vi "lfieldpanel_plot_sensor_data.vi"(7 "Integrate":bool, 8 "error in (no error)":errorcluster, 9 "First_time?":bool, 10 "image_data":T1, 11 "lightfield_panel in":refnum<class "lightfield_panel.lvclass">) -> (0 "error out":errorcluster, 3 "lightfield_panel out":refnum<class "lightfield_panel.lvclass">)   [LabVIEW 2015, in "lightfield_panel.lvclass"]
uses:
  lightfield_panel.lvclass
  UI/panel_class/panel.lvclass/panel.ctl
  <vilib>/Analysis/1siggen.llb/Ramp Pattern by Samples.vi
  UI/panel_class/panel.lvclass
  <vilib>/Analysis/NI_AALBase.lvlib
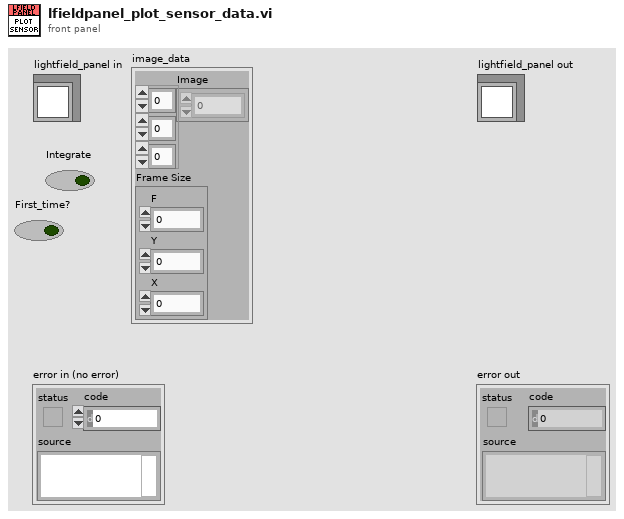
[diagram p1: front panel]
types:
  T1 = cluster{"Image":dbl[][][], "Frame Size":cluster{"F":i32, "Y":i32, "X":i32}}
  T2 = enum32{"Chart", "Graph", "Map", "XY Graph", "Large Readout"}
  T3 = typedef "ui_plot_references.ctl" = cluster{"plots":refnum<vi>, "chart":refnum<vi>, "graph":refnum<vi>, "map":refnum<vi>, "XY Graph":refnum<vi>}
  T4 = typedef "ui_user_events.ctl" = cluster{"update_xy_graph":refnum<user-event>, "update_graph":refnum<user-event>, "update_chart":refnum<user-event>, "update_map":refnum<user-event>, "event_loop_stop":refnum<user-event>, "keep_map":refnum<user-event>}
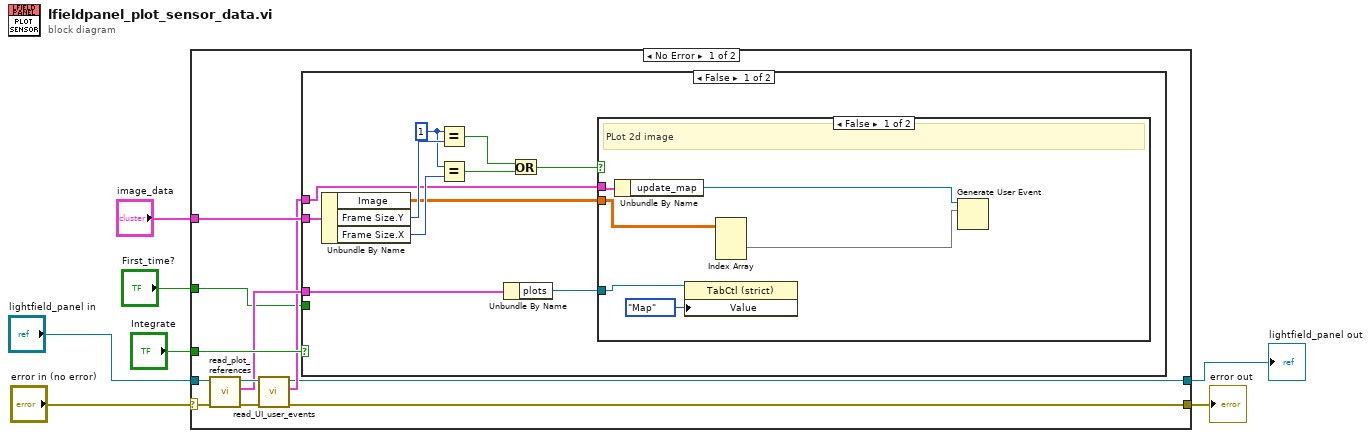
[diagram p0: block diagram]
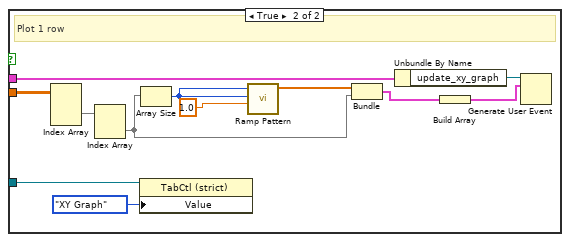
[diagram p2: hidden frame]
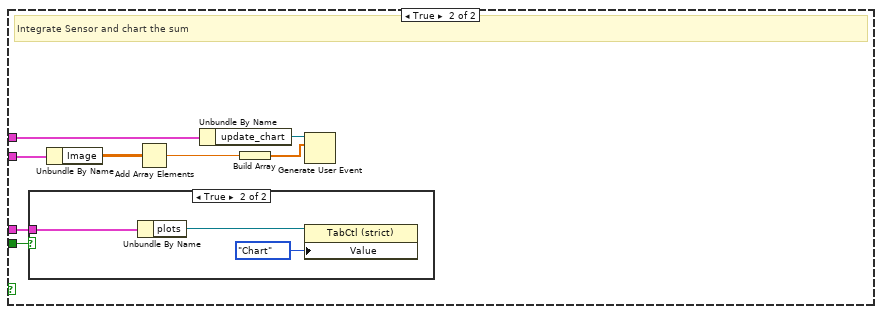
[diagram p3: hidden frame]
diagram:
  n1 = case shown="No Error" "error in (no error)" {
    selector: "error in (no error)" -> [w12 w60]
    tunnel: [w11 w60] -> w6
    tunnel: [w9 w59] -> w4
    tunnel: "lightfield_panel in" -> [w18 w59]
    tunnel: "image_data" -> [w14 _]
    tunnel: "Integrate" -> [w15 _]
    tunnel: "First_time?" -> [w8 _]
    frame No Error {
      n2 = call "read_plot_references.vi"("error in (no error)"=w12, "panel in"=w18) -> ("error out"=w16:errorcluster, "plot_references"=w13:T3, "panel out"=w17:refnum<class "lightfield_panel.lvclass">)  [unwired: 7 in]
      n3 = call "read_UI_user_events.vi"("error in (no error)"=w16, "panel in"=w17) -> ("error out"=w11:errorcluster, "ui_user_events"=w10:T4, "panel out"=w9:refnum<class "lightfield_panel.lvclass">)  [unwired: 7 in]
      n4 = case shown="False" w15 {
        tunnel: w14 -> [w28 w55]
        tunnel: w13 -> [w29 w53]
        tunnel: w10 -> [w20 w51]
        tunnel: w8 -> [_ w52]
        frame False {
          w19 = 1 ("x")
          n5 = Unbundle By Name(w28) -> ("Image"=w21:dbl[][][], "Frame Size.Y"=w27:i32, "Frame Size.X"=w26:i32)
          n6 = Equal?(x=w19, y=w27) -> (x = y?=w25:bool)
          n7 = Equal?(x=w19, y=w26) -> (x = y?=w24:bool)
          n8 = Unbundle By Name(w29) -> ("plots"=w22:refnum<vi>)
          n9 = Or(x=w25, y=w24) -> (x .or. y?=w23:bool)
          n10 = case shown="False" w23 {
            tunnel: w22 -> [w35 w47]
            tunnel: w21 -> [w31 w45]
            tunnel: w20 -> [w33 w43]
            frame False {
              # "PLot 2d image"
              n11 = Unbundle By Name(w33) -> ("update_map"=w32:refnum<user-event>)
              n12 = property class="TabCtl (strict)"(reference=w35, "Value"=T2."Map") -> ()  [unwired: 1 in, 2 out]
              n13 = Index Array(array=w31) -> (element=w30:dbl[][])  [unwired: 3 in]
              n14 = Generate User Event(user event=w32, event data cluster=w30) -> ()  [unwired: 2 in, 2 out]
            }
            frame True {
              # "Plot 1 row"
              n15 = Index Array(array=w45) -> (element=w44:dbl[][])  [unwired: 3 in]
              n16 = Index Array(array=w44) -> (element=w38:dbl[])  [unwired: 2 in]
              n17 = property class="TabCtl (strict)"(reference=w47, "Value"=T2."XY Graph") -> ()  [unwired: 1 in, 2 out]
              n18 = Array Size(array=w38) -> (size(s)=w41:i32)
              n19 = call-poly <vilib>:"Ramp Pattern.vi"("start"=1.0, "end"=w41, "samples"=w41) -> ("Ramp Pattern"=w39:dbl[])  [unwired: 7 in, 1 out]
              n20 = Bundle("Ramp Pattern"=w39, "Image"=w38) -> (w37:cluster{"Ramp Pattern":dbl[], "Image":dbl[]})  [unwired: 1 in]
              n21 = Unbundle By Name(w43) -> ("update_xy_graph"=w42:refnum<user-event>)
              n22 = Build Array(w37) -> (w36:cluster{"Ramp Pattern":dbl[], "Image":dbl[]}[])
              n23 = Generate User Event(user event=w42, event data cluster=w36) -> ()  [unwired: 2 in, 2 out]
            }
          }
        }
        frame True {
          # "Integrate Sensor and chart the sum"
          n24 = case shown="True" w52 {
            tunnel: w53 -> [_ w58]
            frame False {
            }
            frame True {
              n25 = Unbundle By Name(w58) -> ("plots"=w57:refnum<vi>)
              n26 = property class="TabCtl (strict)"(reference=w57, "Value"=T2."Chart") -> ()  [unwired: 1 in, 2 out]
            }
          }
          n27 = Unbundle By Name(w55) -> ("Image"=w54:dbl[][][])
          n28 = Add Array Elements(numeric array=w54) -> (sum=w49:dbl)
          n29 = Unbundle By Name(w51) -> ("update_chart"=w50:refnum<user-event>)
          n30 = Build Array(w49) -> (w48:dbl[])
          n31 = Generate User Event(user event=w50, event data cluster=w48) -> ()  [unwired: 2 in, 2 out]
        }
      }
    }
    frame Error {
    }
  }
  "error out" <- w6
  "lightfield_panel out" <- w4
